vi "WSVCAP SHL Host LL SPI Set Read_Write Parameters.vi"(5 "Wait Ticks":u32, 7 "Elements to Transfer":u8, 9 "Socket Mask [U16]":u16 format="%04x", 11 "error in (no error)":errorcluster) -> (15 "error out":errorcluster)   [LabVIEW 2012]
uses:
  Type Defs/WSVCAP SHL Top Level Control Operation Enum.ctl
  Type Defs/WSVCAP SHL State.ctl
  Type Defs/WSVCAP SHL Top Level Control Enum.ctl
  Type Defs/WSVCAP SHL Transaction Enum.ctl
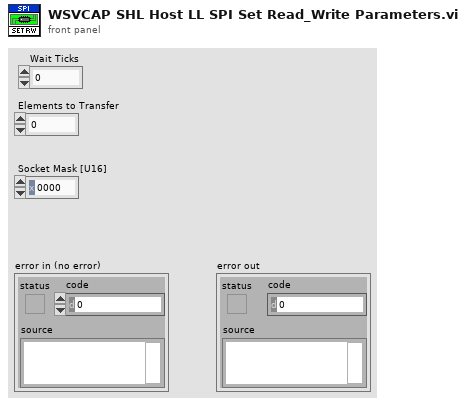
[diagram p1: front panel]
types:
  T1 = typedef "WSVCAP SHL Transaction Enum.ctl" = enum16{"I2C-Read Data", "I2C-Write Data", "SPI-Write/Read Data", "RFFE-Ext Write", "RFFE-Ext Read"}
  T2 = typedef "WSVCAP SHL Top Level Control Enum.ctl" = enum16{"Start", "Cmd", "Transaction", "Wait Ticks", "Socket Mask", "Slave Address", "Sub Address", "Bytes to Write", "Bytes to Read", "Write Data", "Write Flag", "Read Data", "Read Flag", "Ack Read", "Read Status Flag", "Ack Read Status", "Status", "Cycle Count", "Stop Cycle", "Exit"}
  T3 = typedef "WSVCAP SHL State.ctl" = enum8{"Idle", "Transfer Data"}
  T4 = typedef "WSVCAP SHL Top Level Control Operation Enum.ctl" = enum16{"Initialize", "Set Control", "Read Control", "Close"}
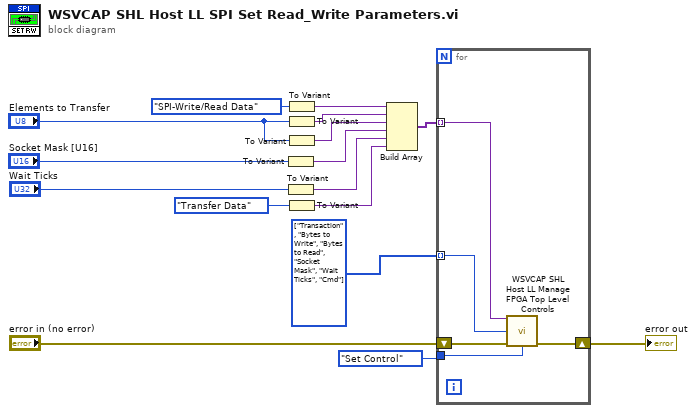
[diagram p0: block diagram]
diagram:
  w8 = T2[] [enum."Transaction", enum."Bytes to Write", enum."Bytes to Read", enum."Socket Mask", enum."Wait Ticks", enum."Cmd"] items=["Start", "Cmd", "Transaction", "Wait Ticks", "Socket Mask", "Slave Address", "Sub Address", "Bytes to Write", "Bytes to Read", "Write Data", "Write Flag", "Read Data", "Read Flag", "Ack Read", "Read Status Flag", "Ack Read Status", "Status", "Cycle Count", "Stop Cycle", "Exit"]
  n1 = To Variant(anything="Socket Mask [U16]") -> (Variant=w4:variant)
  n2 = To Variant(anything="Wait Ticks") -> (Variant=w1:variant)
  n3 = To Variant(anything=WSVCAP_SHL_Transaction_Enum."SPI-Write/Read Data" ("Transaction")) -> (Variant=w14:variant)
  n4 = To Variant(anything="Elements to Transfer") -> (Variant=w13:variant)
  n5 = To Variant(anything="Elements to Transfer") -> (Variant=w7:variant)
  n6 = To Variant(anything=WSVCAP_SHL_State."Transfer Data" ("SPI_Cmd")) -> (Variant=w9:variant)
  n7 = Build Array(w14, w13, w7, w4, w1, w9) -> (w12:variant[])
  n8 = for {
    tunnel: WSVCAP_SHL_Top_Level_Control_Operation_Enum."Set Control" ("Operation") -> [w21]
    tunnel: w12 -> [w20] mode=indexing
    tunnel: w8 -> [w19] mode=indexing
    shift-right: [w17] -> w10
    shift-left: "error in (no error)" -> [w18]
    n9 = call "WSVCAP SHL Host LL Manage FPGA Top Level Controls.vi"("Value In"=w20, "FPGA Top Level Control"=w19, "error in (no error)"=w18, "Operation"=w21) -> ("error out"=w17:errorcluster)  [unwired: 10 in, 1 out]
  }
  "error out" <- w10
